vi "Create VI.vi"(4 "error in":errorcluster, 6 "VI Definition":T1, 7 "Path":path) -> (0 "error out":errorcluster)   [LabVIEW 2025]
doc: "This VI creates a VI according to the provided VI definition in the specified path. This VI sets the description and the VI name as defined and adds the following components: numeric indicators, string controls, free labels, front panel labels and string constants."
uses:
  VI Definition--cluster.ctl
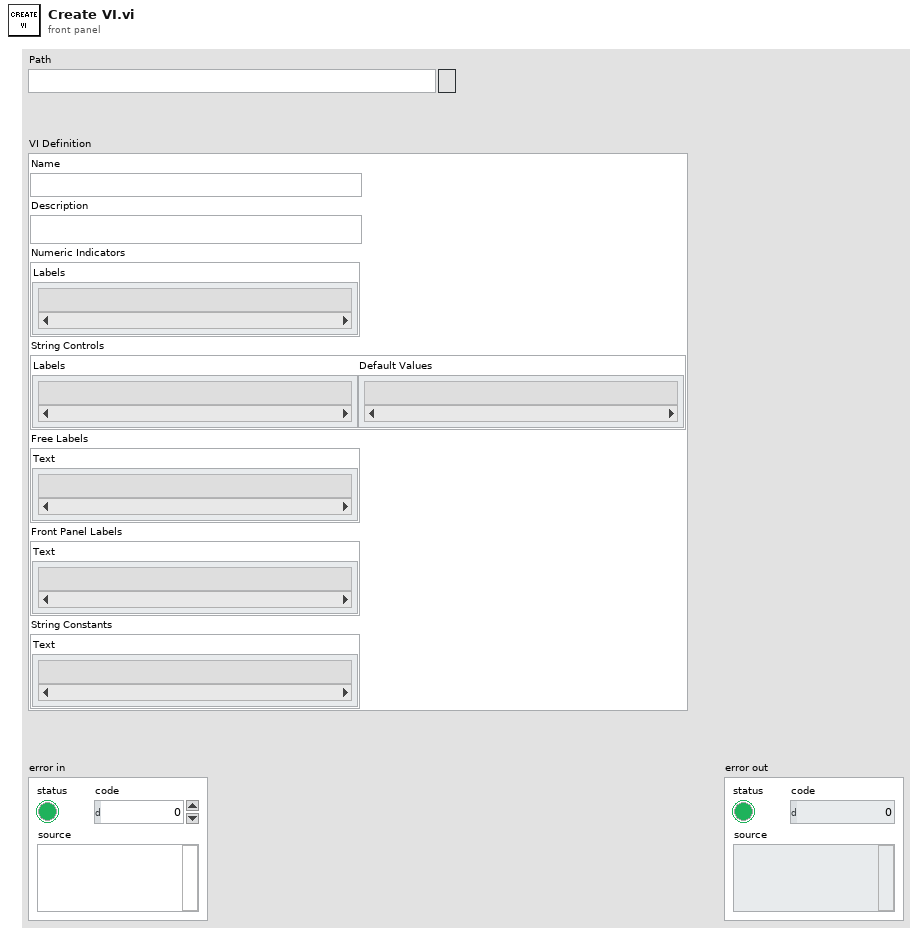
[diagram p1: front panel]
types:
  T1 = typedef "VI Definition--cluster.ctl" = cluster{"Name":string, "Description":string, "Numeric Indicators":cluster{"Labels":string[]}, "String Controls":cluster{"Labels":string[], "Default Values":string[]}, "Free Labels":cluster{"Text":string[]}, "Front Panel Labels":cluster{"Text":string[]}, "String Constants":cluster{"Text":string[]}}
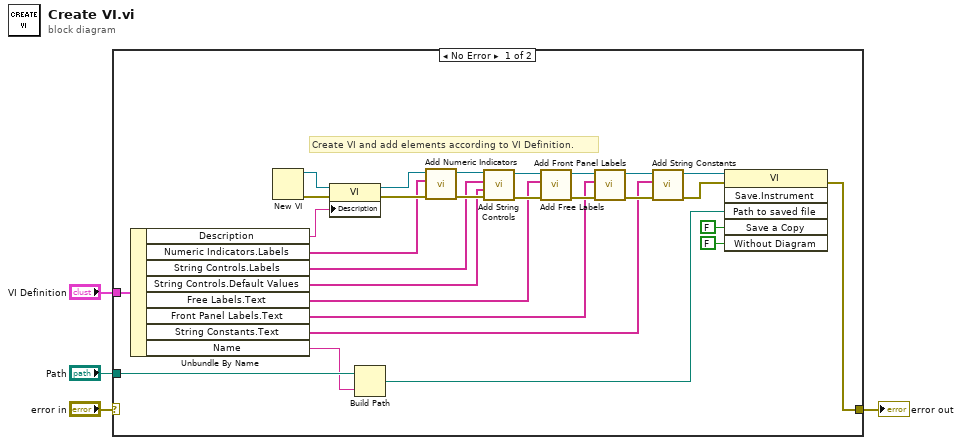
[diagram p0: block diagram]
diagram:
  n1 = case shown="No Error" "error in" {
    selector: "error in" -> [_ w33]
    tunnel: "Path" -> [w19 _]
    tunnel: "VI Definition" -> [w18 _]
    tunnel: [w25 w33] -> w3
    frame No Error {
      # "Create VI and add elements according to VI Definition."
      n2 = Unbundle By Name(w18) -> ("Description"=w9:string, "Numeric Indicators.Labels"=w10:string[], "String Controls.Labels"=w11:string[], "String Controls.Default Values"=w12:string[], "Free Labels.Text"=w13:string[], "Front Panel Labels.Text"=w14:string[], "String Constants.Text"=w15:string[], "Name"=w17:string)
      n3 = New VI() -> (0:w27:errorcluster, 3:w20:refnum<vi>)  [unwired: 7 in]
      n4 = property class="VI"(reference=w20, error in=w27, "Description"=w9) -> (reference out=w5:refnum<vi>, error out=w26:errorcluster)
      n5 = Build Path(base path=w19, name or relative path=w17) -> (appended path=w16:path)
      n6 = call "Add Numeric Indicators.vi"("error in"=w26, "Labels"=w10, "vi refnum"=w5) -> ("error out"=w32:errorcluster, "vi refnum dup"=w7:refnum<vi>)  [unwired: 3 in]
      n7 = call "Add String Controls.vi"("error in"=w32, "Values"=w12, "Labels"=w11, "vi refnum"=w7) -> ("error out"=w31:errorcluster, "vi refnum dup"=w6:refnum<vi>)  [unwired: 2 in]
      n8 = call "Add Free Labels.vi"("error in"=w31, "Labels"=w13, "vi refnum"=w6) -> ("error out"=w30:errorcluster, "vi refnum dup"=w22:refnum<vi>)  [unwired: 3 in]
      n9 = call "Add Front Panel Labels.vi"("error in"=w30, "Labels"=w14, "vi refnum"=w22) -> ("error out"=w29:errorcluster, "vi refnum dup"=w21:refnum<vi>)  [unwired: 3 in]
      n10 = call "Add String Constants.vi"("error in"=w29, "Labels"=w15, "vi refnum"=w21) -> ("error out"=w28:errorcluster, "vi refnum dup"=w8:refnum<vi>)  [unwired: 3 in]
      n11 = invoke class="VI" method="Save.Instrument"(reference=w8, error in=w28, "Path to saved file"=w16, "Save a Copy"=FALSE, "Without Diagram"=FALSE) -> (error out=w25:errorcluster)  [unwired: 1 in, 5 out]
    }
    frame Error {
      # "Pass error without further action"
    }
  }
  "error out" <- w3
